vi "UI Main.vi"() -> ()   [LabVIEW 2014]
panel:
  in  "Stop":bool
  out "VariableIndicator":dbl
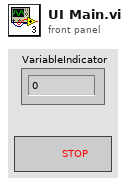
[diagram p1: front panel]
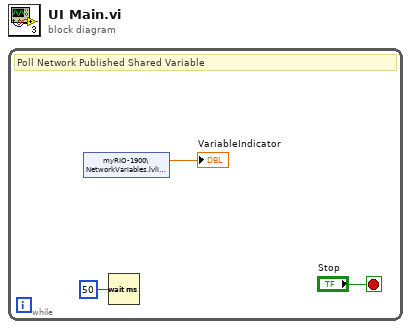
[diagram p0: block diagram]
diagram:
  n1 = while {
    stop <- "Stop" stop-if-true
    # "Poll Network Published Shared Variable"
    n2 = shared-variable "myRIO-1900\\NetworkVariables.lvlib\\variable"() -> (→"VariableIndicator":dbl)  [unwired: 1 in, 1 out]
    n3 = Wait (ms)(milliseconds to wait=u32 50) -> ()  [unwired: 1 out]
  }
